vi "CalVal-Config.vi"(0 "Params In":T1, 11 "error in (no error)":errorcluster) -> (3 "NBuffers":i32, 4 "Params Out":T1, 14 "Mic Avg":dbl[][](array[numeric]), 15 "error out":errorcluster)   [LabVIEW 2020]
uses:
  Type Defs/CalVal-Params.ctl
  epl-vi-lib/Utility VIs/Type Defs/Left-Right ring.ctl
  epl-vi-lib/Connection VIs/Type Defs/Input sources.ctl
  epl-vi-lib/Connection VIs/Type Defs/Output sources.ctl
  epl-vi-lib/Utility VIs/Array Manipulation VIs/Sort and Index (I32).vi
  epl-vi-lib/PXI DAQ VIs/DAQ Engine VIs/AO Gain and Multiplier VIs/PXI Multipliers to AO Gains (1D).vi
panel:
  in  "Buffer length (s)":dbl=0.5
  in  "Attenuation (dB)":dbl=20.0
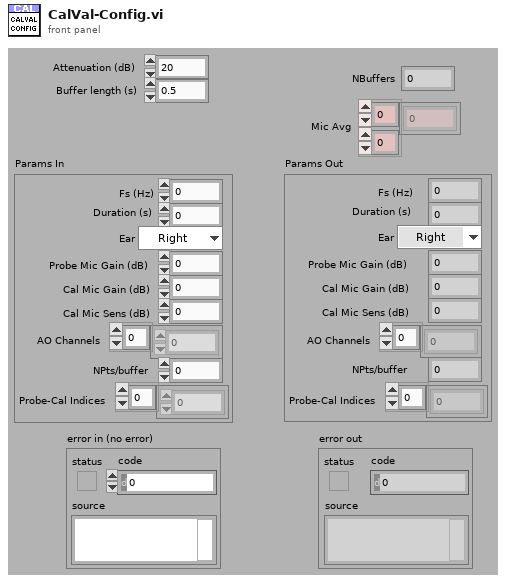
[diagram p1: front panel]
types:
  T1 = typedef "CalVal-Params.ctl" = cluster{"Fs (Hz)":dbl, "Duration (s)":dbl, "Ear":T2, "Probe Mic Gain (dB)":dbl, "Cal Mic Gain (dB)":dbl, "Cal Mic Sens (dB)":dbl, "AO Channels":i32[], "NPts/buffer":i32, "Probe-Cal Indices":i32[]}
  T2 = typedef "Left-Right ring.ctl" = enum16{"Right", "Left"}
  T3 = typedef "Input sources.ctl" = u16
  T4 = typedef "Output sources.ctl" = u16
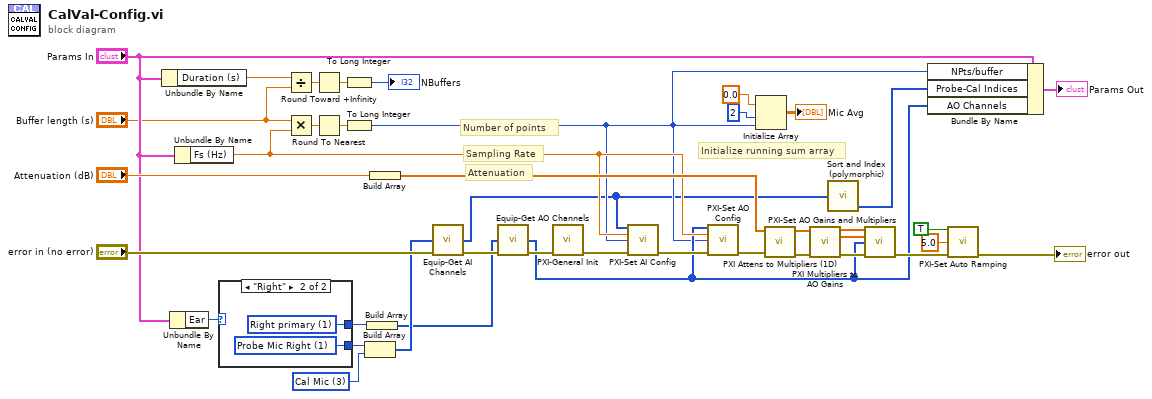
[diagram p0: block diagram]
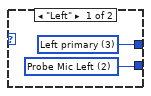
[diagram p2: hidden frame]
diagram:
  w18 = T3 3 items=["--unused--", "Probe Mic Right", "Probe Mic Left", "Cal Mic", "ABR", "CAP Right", "CAP Left", "Startle piezo", "Temperature", "Heart rate"] ("Ring")
  # "Attenuation"
  # "Sampling Rate"
  # "Number of points"
  # "Initialize running sum array"
  n1 = Unbundle By Name("Params In") -> ("Duration (s)"=w8:dbl)
  n2 = Unbundle By Name("Params In") -> ("Ear"=w12:T2)
  n3 = Unbundle By Name("Params In") -> ("Fs (Hz)"=w13:dbl)
  n4 = case shown="\"Right\"" w12 {
    tunnel: [w41 w43] -> w19
    tunnel: [w42 w44] -> w35
    frame "Left" {
      w41 = T4 3 items=["--unused--", "Right primary", "Right secondary", "Left primary", "Left secondary", "Shocks", "Startle", "Background"] ("Ring")
      w42 = T3 2 items=["--unused--", "Probe Mic Right", "Probe Mic Left", "Cal Mic", "ABR", "CAP Right", "CAP Left", "Startle piezo", "Temperature", "Heart rate"] ("Ring")
    }
    frame "Right" {
      w43 = T4 1 items=["--unused--", "Right primary", "Right secondary", "Left primary", "Left secondary", "Shocks", "Startle", "Background"] ("Ring")
      w44 = T3 1 items=["--unused--", "Probe Mic Right", "Probe Mic Left", "Cal Mic", "ABR", "CAP Right", "CAP Left", "Startle piezo", "Temperature", "Heart rate"] ("Ring")
    }
  }
  n5 = Divide(x=w8, y="Buffer length (s)") -> (x/y=w6:dbl)
  n6 = Multiply(x="Buffer length (s)", y=w13) -> (x*y=w34:dbl)
  n7 = Round Toward +Infinity(x=w6) -> (ceil(x): smallest int >= x=w5:dbl)
  n8 = Round To Nearest(number=w34) -> (nearest integer value=w33:dbl)
  n9 = To Long Integer(number=w5) -> (32bit integer=→"NBuffers":i32)
  n10 = To Long Integer(number=w33) -> (32bit integer=w3:i32)
  n11 = Build Array(w35, w18) -> (w31:T3[])
  n12 = Build Array(w19) -> (w15:T4[])
  n13 = Build Array("Attenuation (dB)") -> (w14:dbl[])
  n14 = call "Equip-Get AI Channels.vi"("Inputs"=w31, "error in (no error)"="error in (no error)") -> ("AI Channels"=w2:i32[], "error out"=w21:errorcluster)  [unwired: 12 in]
  n15 = call "Equip-Get AO Channels.vi"("Outputs"=w15, "error in (no error)"=w21) -> ("AO Channels"=w11:i32[], "error out"=w16:errorcluster)  [unwired: 12 in]
  n16 = call "PXI-General Init.vi"("error in (no error)"=w16) -> ("error out"=w30:errorcluster)  [unwired: 10 in]
  n17 = call "PXI-Set AI Config.vi"("AI Channels"=w2, "Sampling Rate (Hz)"=w13, "Buffer Size"=w3, "error in (no error)"=w30) -> ("error out"=w29:errorcluster)  [unwired: 11 in]
  n18 = call "PXI-Set AO Config.vi"("AO Channels"=w11, "Sampling Rate (Hz)"=w13, "Buffer Size"=w3, "error in (no error)"=w29) -> ("error out"=w28:errorcluster)  [unwired: 11 in]
  n19 = Initialize Array(0.0 ("element"), 2 ("dimension size"), w3) -> (→"Mic Avg":dbl[][])
  n20 = call "PXI Attens to Multipliers (1D).vi"("error in (no error)"=w28, "Array of Attens"=w14) -> ("error out"=w40:errorcluster, "Multiplier setting"=w39:dbl[])  [unwired: 8 in]
  n21 = call-poly "PXI Multipliers to AO Gains.vi"("Multipliers in"=w39, "error in (no error)"=w40) -> ("Multipliers out"=w26:dbl[], "Gains"=w24:dbl[], "error out"=w27:errorcluster)  [unwired: 11 in]
  n22 = call-poly "Sort and Index (polymorphic).vi"("X"=w2) -> ("Index"=w1:i32[])  [unwired: 3 in, 1 out]
  n23 = call "PXI-Set AO Gains and Multipliers.vi"("Multipliers"=w26, "Gains"=w24, "AO Channels"=w11, "error in (no error)"=w27) -> ("error out"=w25:errorcluster)  [unwired: 11 in]
  n24 = Bundle By Name(cluster="Params In", "NPts/buffer"=w3, "Probe-Cal Indices"=w1, "AO Channels"=w11) -> (→"Params Out":T1)
  n25 = call "PXI-Set Auto Ramping.vi"("Auto ramp?"=TRUE, "Ramp duration (ms)"=5.0, "error in (no error)"=w25) -> ("error out"=→"error out":errorcluster)  [unwired: 12 in]
